vi "CIF Template UI.vi"() -> ()   [LabVIEW 2021, in "CIF Template UI.lvlib"]
uses:
  CIF Template UI.lvlib
  CIF-LVCore/src/CIFUI/Typedef/Channel Connection.ctl
  CIF-LVCore/src/CIFUI/Typedef/Force Channel.ctl
  CIF-LVCore/src/CIFUI/Typedef/Run Listen Button.ctl
  Common/Typedef/Configuration.ctl
  CIF-LVCore/src/CIFCore/Common/Typedef/Common Plugin Configuration.ctl
  CIF-LVCore/src/CIFUI/Typedef/Core UI References.ctl
  CIF-LVCore/src/CIFUI/CIF_UI.lvclass/CIF_UI.ctl
  CIF-LVCore/src/CIFUI/Typedef/Direction to Include.ctl
  CIF-LVCore/src/CIFUI/UI Element Update/Empty Tree.vi
  CIF-LVCore/src/CIFUI/UI Element Update/Empty Table.vi
  CIF-LVCore/src/CIFUI/CIF_UI.lvclass
  <vilib>/addons/_JKI.lib/Serialization/JSON/JKI JSON Serialization.lvlib
  Grpc/Template_wrapper/TemplateWrapper.lvlib
  CIF-LVCore/src/CIFCore/Common/CIFCoreCommon.lvlib
  Common/TemplateCommon.lvlib
panel:
  in  "Plugin Status":string[][](table)
  in  "Configuration":T1={"Common"={"Period (s)"=0.001, "Offset (us)"=0, "ClockID"=0, "Priority"=100, "Processor"=-2}, "Step"=100} {"Common"."Period (s)" format="%#_13g"}
  out "Errors":string
  in  "Run Listen":T3
  in  "Exit":bool
  out "Connected":bool
  in  "Connection":bool
  in  "Force Channel":T4
  in  "Link Channel":bool
  in  "Connection":T5
  in  "Channels":string(tree)
  in  "address":string="192.168.1.160"
  in  "Clear Local":bool
  in  "Force":bool
  in  "Unload":bool
  in  "Refresh Button":bool
  in  "Update Config":bool
  in  "Session Id":u64
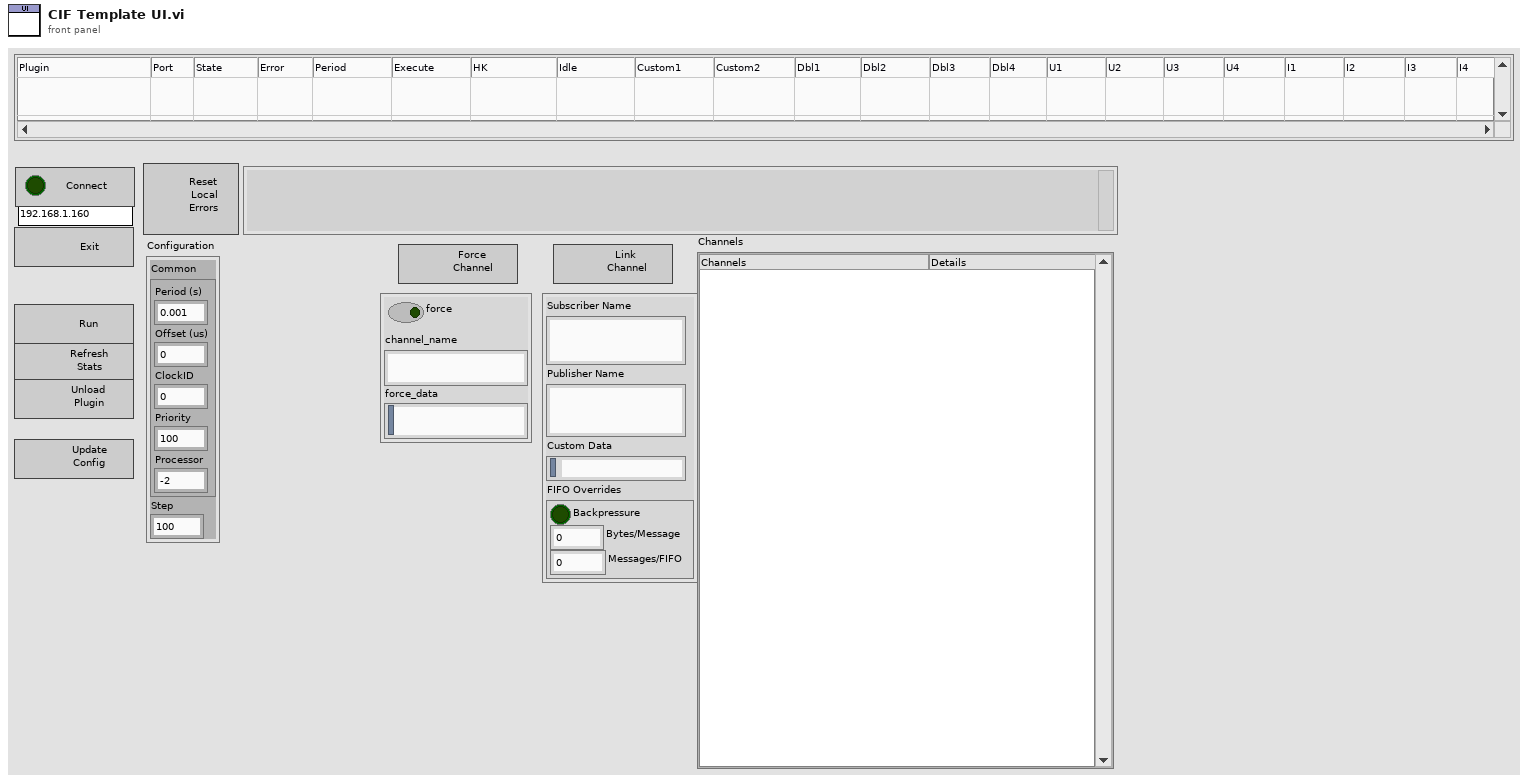
[diagram p1: front panel]
types:
  T1 = typedef "TemplateCommon.lvlib/Configuration.ctl" = cluster{"Common":T2, "Step":u64}
  T2 = typedef "CIFCoreCommon.lvlib/Common Plugin Configuration.ctl" = cluster{"Period (s)":dbl, "Offset (us)":i32, "ClockID":u8, "Priority":i32, "Processor":i32}
  T3 = typedef "CIF_UI.lvclass/Run Listen Button.ctl" = bool
  T4 = typedef "CIF_UI.lvclass/Force Channel.ctl" = cluster{"channel_name":string, "force":bool, "force_data":string}
  T5 = typedef "CIF_UI.lvclass/Channel Connection.ctl" = cluster{"Subscriber Name":string, "Publisher Name":string, "Custom Data":string, "FIFO Overrides":cluster{"Backpressure":bool, "Bytes/Message":u32, "Messages/FIFO":u32}}
  T6 = typedef "CIF_UI.lvclass/Core UI References.ctl" = cluster{"Discovered Plugins":refnum<vi>, "Discovered Plugins Valid":bool, "Loaded Plugins":refnum<vi>, "Loaded Plugins Valid":bool, "Publisher Channels":refnum<vi>, "Publisher Channels Valid":bool, "Subscriber Channels":refnum<vi>, "Subscriber Channels Valid":bool, "Plugin Status":refnum<vi>, "Plugin Status Valid":bool, "Channel Connection":refnum<vi>, "Channel Connection Valid":bool, "New Plugin Load":refnum<vi>, "New Plugin Load Valid":bool, "Errors":refnum<vi>, "Errors Valid":bool, "Plugin to Abort":refnum<vi>, "Plugin to Abort Valid":bool, "Connection":refnum<vi>, "Connection Valid":bool, "Exit":refnum<vi>, "Exit Valid":bool, "Run Listen":refnum<vi>, "Run Listen Valid":bool}
  T7 = typedef "InstrumentStudio Plugin SDK.lvlib/Event Registration Refnum.ctl" = refnum<event-registration>
  T8 = typedef "CIF_UI.lvclass/Direction to Include.ctl" = enum16{"All", "Subscriber", "Publisher"}
  T9 = typedef "grpc-lvsupport-release.lvlib/grpcId.ctl" = u64
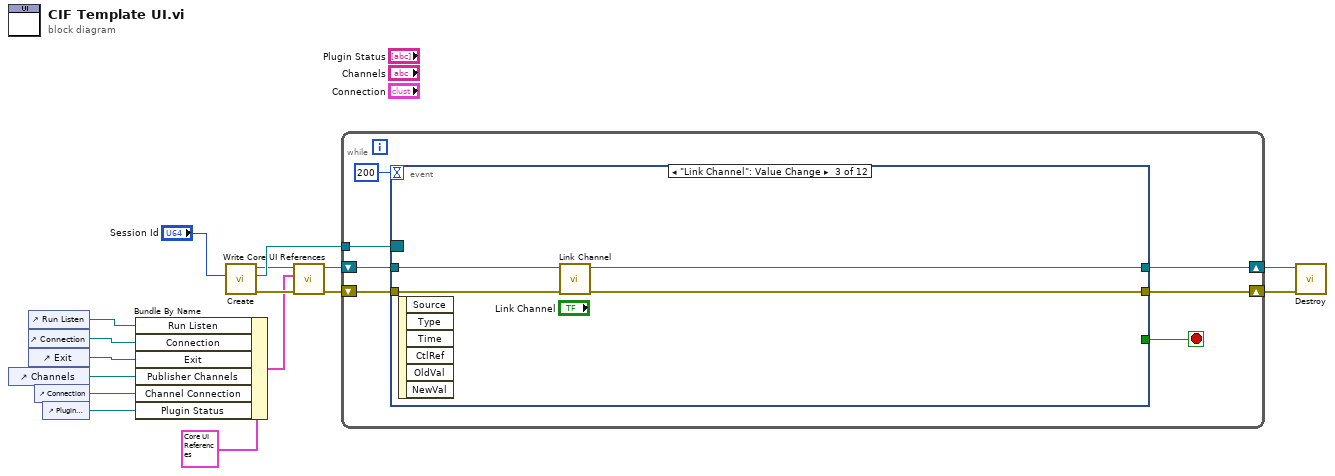
[diagram p0: block diagram]
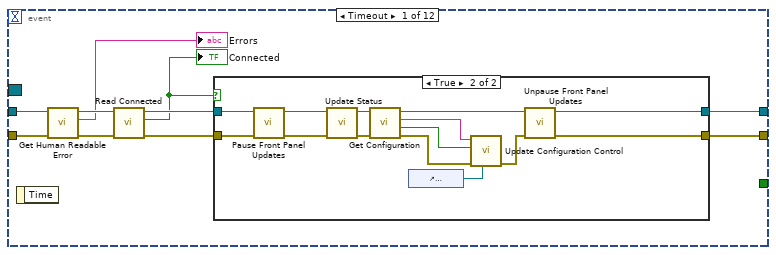
[diagram p2: hidden frame]
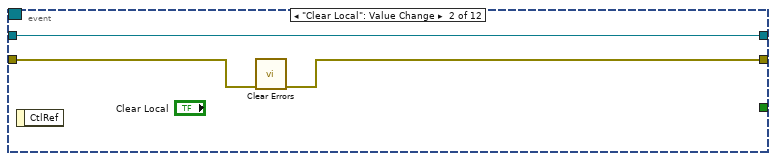
[diagram p4: hidden frame]
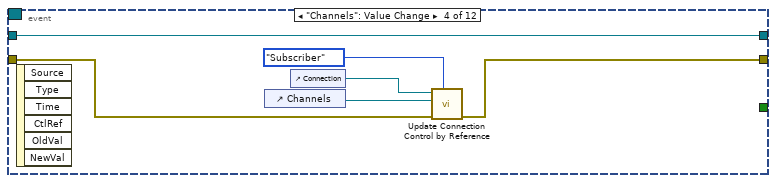
[diagram p5: hidden frame]
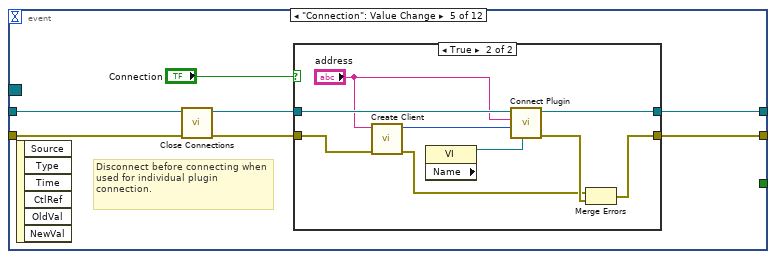
[diagram p6: hidden frame]
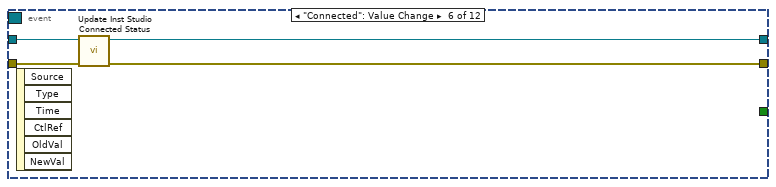
[diagram p8: hidden frame]
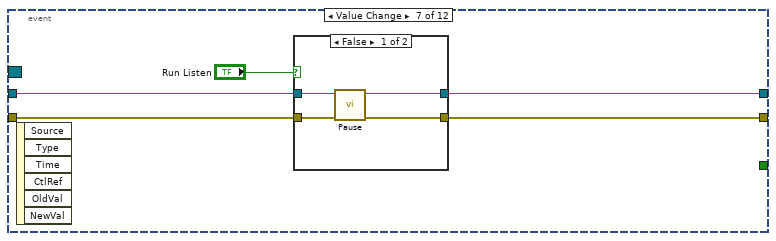
[diagram p9: hidden frame]
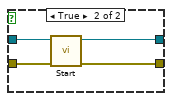
[diagram p10: hidden frame]
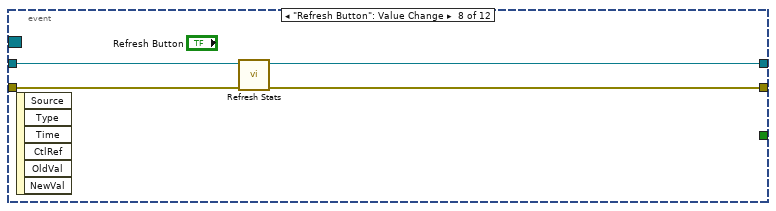
[diagram p11: hidden frame]
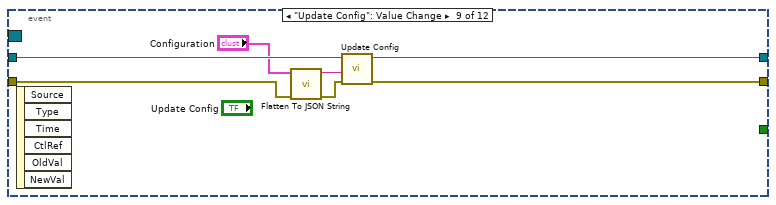
[diagram p12: hidden frame]
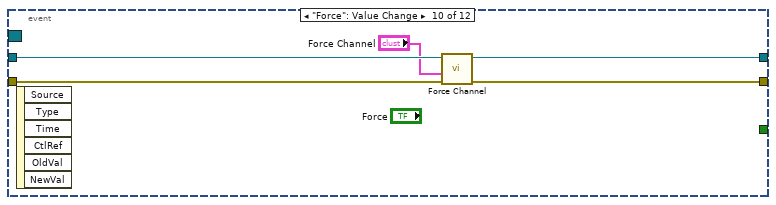
[diagram p13: hidden frame]
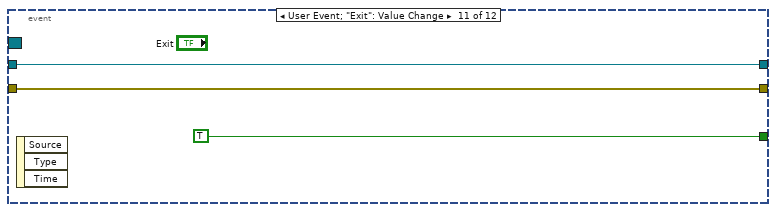
[diagram p14: hidden frame]
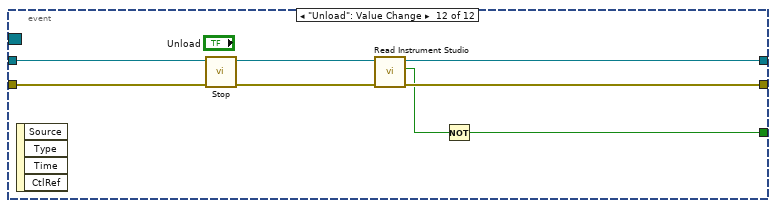
[diagram p15: hidden frame]
diagram:
  n1 = control-ref of="Channels"() -> (w14:refnum<vi>)
  n2 = control-ref of="Run Listen"() -> (w3:refnum<vi>)
  n3 = control-ref of="Connection"() -> (w4:refnum<vi>)
  n4 = control-ref of="Exit"() -> (w5:refnum<vi>)
  n5 = control-ref of="Connection"() -> (w2:refnum<vi>)
  n6 = control-ref of="Plugin Status"() -> (w1:refnum<vi>)
  n7 = Bundle By Name(cluster=T6 {"Discovered Plugins"=refnum, "Discovered Plugins Valid"=FALSE, "Loaded Plugins"=refnum, "Loaded Plugins Valid"=FALSE, "Publisher Channels"=refnum, "Publisher Channels Valid"=FALSE, "Subscriber Channels"=refnum, "Subscriber Channels Valid"=FALSE, "Plugin Status"=refnum, "Plugin Status Valid"=FALSE, "Channel Connection"=refnum, "Channel Connection Valid"=FALSE, "New Plugin Load"=refnum, "New Plugin Load Valid"=FALSE, "Errors"=refnum, "Errors Valid"=FALSE, "Plugin to Abort"=refnum, "Plugin to Abort Valid"=FALSE, "Connection"=refnum, "Connection Valid"=FALSE, "Exit"=refnum, "Exit Valid"=FALSE, "Run Listen"=refnum, "Run Listen Valid"=FALSE} ("UI References"), "Run Listen"=w3, "Connection"=w4, "Exit"=w5, "Publisher Channels"=w14, "Channel Connection"=w2, "Plugin Status"=w1) -> (w7:T6)
  n8 = call "Create.vi"("Session Id"="Session Id") -> ("error out"=w10:errorcluster, "Event Refnum"=w13:T7, "CIF_UI out"=w11:refnum<class "CIF_UI.lvclass">)  [unwired: 8 in]
  n9 = call "Write Core UI References.vi"("error in (no error)"=w10, "UI References"=w7, "CIF_UI in"=w11) -> ("error out"=w8:errorcluster, "CIF_UI out"=w9:refnum<class "CIF_UI.lvclass">)  [unwired: 7 in]
  n10 = while {
    tunnel: w13 -> [w22]
    shift-right: [w17] -> w15
    shift-left: w9 -> [w20]
    shift-right: [w18] -> w16
    shift-left: w8 -> [w19]
    stop <- w21 stop-if-true
    n11 = event shown="[2] \"Link Channel\": Value Change" {
      selector: w22 -> [_ _ _ _ _ _ _ _ _ _ _ _]
      dyn-events: _ -> [_ _ _ _ _ _ _ _ _ _ _ _]
      timeout: 200 -> [_ _ _ _ _ _ _ _ _ _ _ _]
      tunnel: [_ _ _ _ _ _ _ _ _ _ TRUE w117] -> w21
      tunnel: w20 -> [w27 w50 w56 w57 w67 w84 w88 w101 w108 w113 w115 w124]
      tunnel: w19 -> [w28 w52 w55 w59 w66 w83 w89 w100 w104 w112 w114 w123]
      tunnel: [w29 w51 w54 w58 w69 w82 w86 w99 w106 w110 w114 w119] -> w18
      tunnel: [w33 w50 w53 w57 w68 w81 w87 w98 w107 w111 w115 w120] -> w17
      event Timeout {
        n12 = event-data() -> ()  [unwired: 1 in, 1 out]
        n13 = call "Get Human Readable Error.vi"("error in (no error)"=w28, "CIF_UI in"=w27) -> ("error out"=w26:errorcluster, "Error Message"=→"Errors":string, "CIF_UI out"=w25:refnum<class "CIF_UI.lvclass">)  [unwired: 7 in]
        n14 = call "Read Connected.vi"("error in (no error)"=w26, "CIF_UI in"=w25) -> ("error out"=w31:errorcluster, "Connected"=w30:bool, "CIF_UI out"=w32:refnum<class "CIF_UI.lvclass">)  [unwired: 7 in]
        "Connected" <- w30
        n15 = case shown="True" w30 {
          tunnel: w31 -> [w34 w46]
          tunnel: [w34 w49] -> w29
          tunnel: w32 -> [w35 w47]
          tunnel: [w35 w48] -> w33
          frame False {
          }
          frame True {
            n16 = call "Pause Front Panel Updates.vi"("error in (no error)"=w46, "CIF_UI in"=w47) -> ("error out"=w45:errorcluster, "CIF_UI out"=w44:refnum<class "CIF_UI.lvclass">)  [unwired: 8 in]
            n17 = call "Update Status.vi"("error in (no error)"=w45, "CIF_UI in"=w44) -> ("error out"=w42:errorcluster, "CIF_UI out"=w43:refnum<class "CIF_UI.lvclass">)  [unwired: 8 in]
            n18 = call "Get Configuration.vi"("error in (no error)"=w42, "CIF_Plugin_UI in"=w43) -> ("error out"=w40:errorcluster, "Not Found"=w37:bool, "JSON Configuration"=w38:string, "CIF_Plugin_UI out"=w41:refnum<class "CIF_UI.lvclass">)  [unwired: 6 in]
            n19 = control-ref of="Configuration"() -> (w36:refnum<vi>)
            n20 = call "Update Configuration Control.vi"("Configuration reference"=w36, "error in (no error)"=w40, "Not Valid"=w37, "JSON Configuration"=w38) -> ("error out"=w39:errorcluster)  [unwired: 7 in]
            n21 = call "Unpause Front Panel Updates.vi"("error in (no error)"=w39, "CIF_UI in"=w41) -> ("error out"=w49:errorcluster, "CIF_UI out"=w48:refnum<class "CIF_UI.lvclass">)  [unwired: 8 in]
          }
        }
      }
      event "Clear Local": Value Change {
        n22 = event-data() -> ()  [unwired: 1 in, 1 out]
        n23 = call <vilib>:"Clear Errors.vi"("error in (no error)"=w52) -> ("error out"=w51:errorcluster)  [unwired: 5 in, 1 out]
      }
      event "Link Channel": Value Change {
        n24 = event-data() -> ()  [unwired: 1 in, 6 out]
        n25 = call "Link Channel.vi"("error in (no error)"=w55, "CIF_UI in"=w56) -> ("error out"=w54:errorcluster, "CIF_UI out"=w53:refnum<class "CIF_UI.lvclass">)  [unwired: 8 in]
      }
      event "Channels": Value Change {
        n26 = event-data() -> ()  [unwired: 1 in, 6 out]
        n27 = control-ref of="Channels"() -> (w60:refnum<vi>)
        n28 = control-ref of="Connection"() -> (w61:refnum<vi>)
        n29 = call "Update Connection Control by Reference.vi"("Direction to Include"=Direction_to_Include."Subscriber", "error in (no error)"=w59, "Channels"=w60, "Channel Connection"=w61) -> ("error out"=w58:errorcluster)  [unwired: 7 in]
      }
      event "Connection": Value Change {
        # "Disconnect before connecting when used for individual plugin connection."
        n30 = event-data() -> ()  [unwired: 1 in, 6 out]
        n31 = call "Close Connections.vi"("error in (no error)"=w66, "CIF_UI in"=w67) -> ("error out"=w64:errorcluster, "CIF_UI out"=w65:refnum<class "CIF_UI.lvclass">)  [unwired: 8 in]
        n32 = case shown="True" "Connection" {
          tunnel: [w70 w80] -> w69
          tunnel: [w71 w78] -> w68
          tunnel: w65 -> [w71 w77]
          tunnel: w64 -> [w70 w76]
          frame False {
          }
          frame True {
            n33 = call "Create Client.vi"("error in"=w76, "address"="address") -> ("error out"=w75:errorcluster, "gRPC ID Out"=w72:T9)  [unwired: 8 in]
            n34 = property class="VI" props=["Name"]() -> (reference out=w73:refnum<vi>)  [unwired: 2 in, 2 out]
            n35 = call "Connect Plugin.vi"("VI Reference"=w73, "gRPC ID"=w72, "Address"="address", "CIF_UI in"=w77) -> ("error out"=w79:errorcluster, "CIF_UI out"=w78:refnum<class "CIF_UI.lvclass">)  [unwired: 6 in]
            n36 = Merge Errors(w75, w79) -> (w80:errorcluster)
          }
        }
      }
      event "Connected": Value Change {
        n37 = event-data() -> ()  [unwired: 1 in, 6 out]
        n38 = call "Update Inst Studio Connected Status.vi"("error in (no error)"=w83, "CIF_UI in"=w84) -> ("error out"=w82:errorcluster, "CIF_UI out"=w81:refnum<class "CIF_UI.lvclass">)  [unwired: 8 in]
      }
      event Value Change {
        n39 = event-data() -> ()  [unwired: 1 in, 6 out]
        n40 = case shown="False" "Run Listen" {
          tunnel: w89 -> [w93 w97]
          tunnel: w88 -> [w92 w96]
          tunnel: [w90 w95] -> w87
          tunnel: [w91 w94] -> w86
          frame False {
            n41 = call "Pause.vi"("error in (no error)"=w93, "CIF_Plugin_UI in"=w92) -> ("error out"=w91:errorcluster, "CIF_Plugin_UI out"=w90:refnum<class "CIF_UI.lvclass">)  [unwired: 7 in, 1 out]
          }
          frame True {
            n42 = call "Start.vi"("error in (no error)"=w97, "CIF_Plugin_UI in"=w96) -> ("error out"=w94:errorcluster, "CIF_Plugin_UI out"=w95:refnum<class "CIF_UI.lvclass">)  [unwired: 7 in, 1 out]
          }
        }
      }
      event "Refresh Button": Value Change {
        n43 = event-data() -> ()  [unwired: 1 in, 6 out]
        n44 = call "Refresh Stats.vi"("error in (no error)"=w100, "CIF_Plugin_UI in"=w101) -> ("error out"=w99:errorcluster, "CIF_Plugin_UI out"=w98:refnum<class "CIF_UI.lvclass">)  [unwired: 7 in, 1 out]
      }
      event "Update Config": Value Change {
        n45 = event-data() -> ()  [unwired: 1 in, 6 out]
        n46 = call <vilib>:"Flatten To JSON String.vi"("error in (no error)"=w104, "Variant"="Configuration") -> ("error out"=w102:errorcluster, "JSON String"=w103:string)  [unwired: 8 in]
        n47 = call "Update Config.vi"("error in (no error)"=w102, "JSON Configuration"=w103, "CIF_Plugin_UI in"=w108) -> ("error out"=w106:errorcluster, "CIF_Plugin_UI out"=w107:refnum<class "CIF_UI.lvclass">)  [unwired: 6 in, 1 out]
      }
      event "Force": Value Change {
        n48 = event-data() -> ()  [unwired: 1 in, 6 out]
        n49 = call "Force Channel.vi"("error in (no error)"=w112, "Force Channel"="Force Channel", "CIF_Plugin_UI in"=w113) -> ("error out"=w110:errorcluster, "CIF_Plugin_UI out"=w111:refnum<class "CIF_UI.lvclass">)  [unwired: 6 in, 1 out]
      }
      event User Event; "Exit": Value Change {
        n50 = event-data() -> ()  [unwired: 1 in, 3 out]
      }
      event "Unload": Value Change {
        n51 = event-data() -> ()  [unwired: 1 in, 4 out]
        n52 = call "Stop.vi"("error in (no error)"=w123, "CIF_Plugin_UI in"=w124) -> ("error out"=w121:errorcluster, "CIF_Plugin_UI out"=w122:refnum<class "CIF_UI.lvclass">)  [unwired: 7 in, 1 out]
        n53 = call "Read Instrument Studio.vi"("error in (no error)"=w121, "CIF_UI in"=w122) -> ("error out"=w119:errorcluster, "Instrument Studio"=w118:bool, "CIF_UI out"=w120:refnum<class "CIF_UI.lvclass">)  [unwired: 7 in]
        n54 = Not(x=w118) -> (.not. x?=w117:bool)
      }
    }
  }
  n55 = call "Destroy.vi"("error in (no error)"=w16, "CIF_UI in"=w15) -> ()  [unwired: 8 in, 2 out]
